vi "agilent_test_3.vi"() -> ()   [LabVIEW 2016]
uses:
  <instrlib>/Keysight PNA Series/Keysight PNA Series.lvlib
panel:
  out "Self-Test Result Code":i32
  out "Self-Test Result Message":string
  out "error out":errorcluster
  in  "VISA resource name":refnum<visa-resource-name>="vna"
  in  "error in (no error)":errorcluster
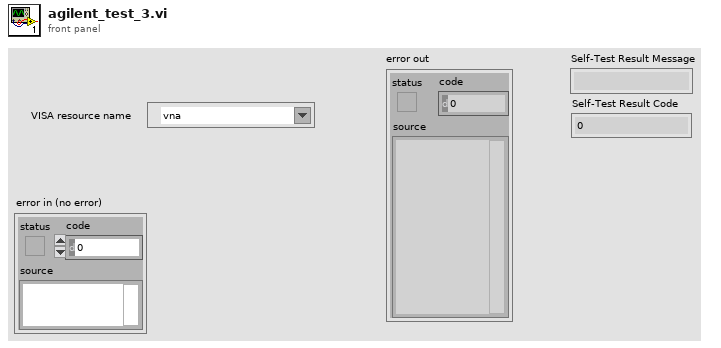
[diagram p1: front panel]
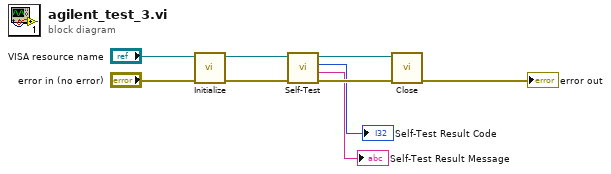
[diagram p0: block diagram]
diagram:
  n1 = call <instrlib>:"Initialize.vi"("error in (no error)"="error in (no error)", "VISA resource name"="VISA resource name") -> ("error out"=w6:errorcluster, "VISA resource name out"=w5:refnum<visa-resource-name>)  [unwired: 8 in]
  n2 = call <instrlib>:"Self-Test.vi"("error in (no error)"=w6, "VISA resource name"=w5) -> ("error out"=w3:errorcluster, "Self-Test Result Message"=→"Self-Test Result Message":string, "Self-Test Result Code"=→"Self-Test Result Code":i32, "VISA resource name out"=w4:refnum<visa-resource-name>)  [unwired: 6 in]
  n3 = call <instrlib>:"Close.vi"("error in (no error)"=w3, "VISA resource name"=w4) -> ("error out"=→"error out":errorcluster)  [unwired: 9 in]
